vi "_Create AnalogIn.vi"(8 "error in (no error)":errorcluster, 10 "ADC #":T1=-1, 11 "Session in":refnum<class "Session.lvclass">) -> (0 "error out":errorcluster, 2 "AnalogIn out":refnum<class "AI.lvclass">, 3 "Session out":refnum<class "Session.lvclass">)   [LabVIEW 2020, in "CTI.lvlib" / "Session.lvclass"]
uses:
  Session.lvclass
  Session.lvclass/Session.ctl
  GPIO/GPIO.lvclass
  Resource/Resource.lvclass
  AI/AI.lvclass
  ADC Number.ctl
  CTI.lvlib
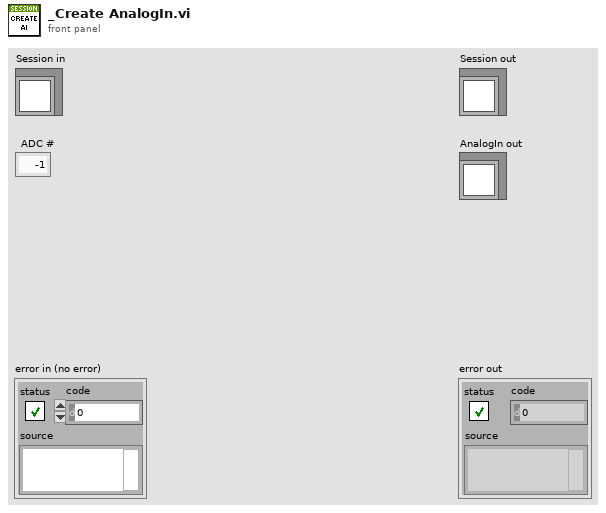
[diagram p1: front panel]
types:
  T1 = typedef "CTI.lvlib/ADC Number.ctl" = i8
  T2 = typedef "CTI.lvlib/GPIO Number.ctl" = i8
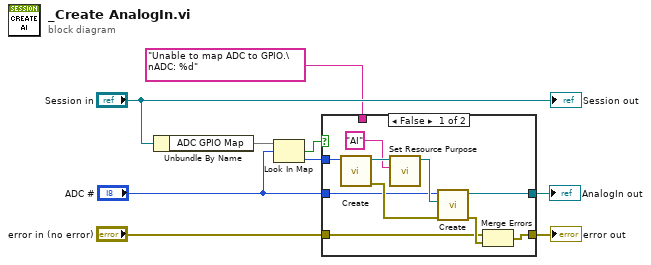
[diagram p0: block diagram]
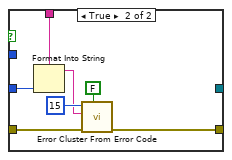
[diagram p2: hidden frame]
diagram:
  n1 = Unbundle By Name("Session in") -> ("ADC GPIO Map"=w9:map{T1, T2})
  n2 = Look In Map(map=w9, key="ADC #") -> (key not found?=w7:bool, value=w8:T2)  [unwired: 1 in]
  n3 = case shown="False" w7 {
    tunnel: w8 -> [w18 _]
    tunnel: [w12 w26] -> w2
    tunnel: "ADC #" -> [w15 w23]
    tunnel: "Unable to map ADC to GPIO.\nADC: %d" -> [_ w22]
    tunnel: "error in (no error)" -> [w11 w20]
    tunnel: [w10 _] -> w1
    frame False {
      n4 = call "Create.vi"("GPIO #"=w18) -> ("error out"=w19:errorcluster, "GPIO out"=w17:refnum<class "GPIO.lvclass">)  [unwired: 9 in]
      n5 = call "Set Resource Purpose.vi"("Resource Purpose"="AI", "Resource in"=w17) -> ("Resource out"=w16:refnum<class "GPIO.lvclass">)  [unwired: 9 in]
      n6 = call "Create.vi"("error in (no error)"=w19, "GPIO"=w16, "ADC #"=w15) -> ("error out"=w13:errorcluster, "AnalogIn out"=w10:refnum<class "AI.lvclass">)  [unwired: 7 in]
      n7 = Merge Errors(w11, w13) -> (w12:errorcluster)
    }
    frame True {
      n8 = Format Into String(format string=w22, w23) -> (resulting string=w21:string)  [unwired: 2 in, 1 out]
      n9 = call <vilib>:"Error Cluster From Error Code.vi"("show call chain? (False)"=FALSE, "error in (no error)"=w20, "error message (\"\")"=w21, "error code (0)"=15) -> ("error out"=w26:errorcluster)  [unwired: 5 in]
    }
  }
  "error out" <- w2
  "AnalogIn out" <- w1
  "Session out" <- "Session in"
